vi "test_null_map.vi"() -> ()   [LabVIEW 2009]
doc: "Copyright (C) 2009, Stepan A. Baranov\nweb: http://www.OCTLab.org/\nemail: stepan@baranov.su"
uses:
  OCTLib.dll
panel:
  out "error out":errorcluster
  out "radius":i32
  out "width":i32
  out "height":i32
  in  "Small/Big":bool
  out "loop #":i32
  out "RSM_STAT time":u32
  out "LabView time":u32
  out "RSM_STAT Array":dbl[][](array[numeric])
  out "LabView Array":dbl[][](array[numeric])
  in  "stop":bool
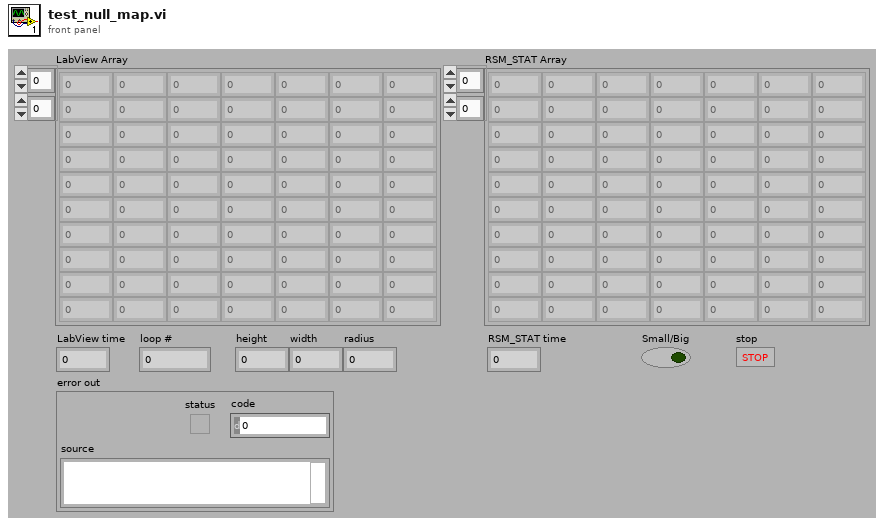
[diagram p1: front panel]
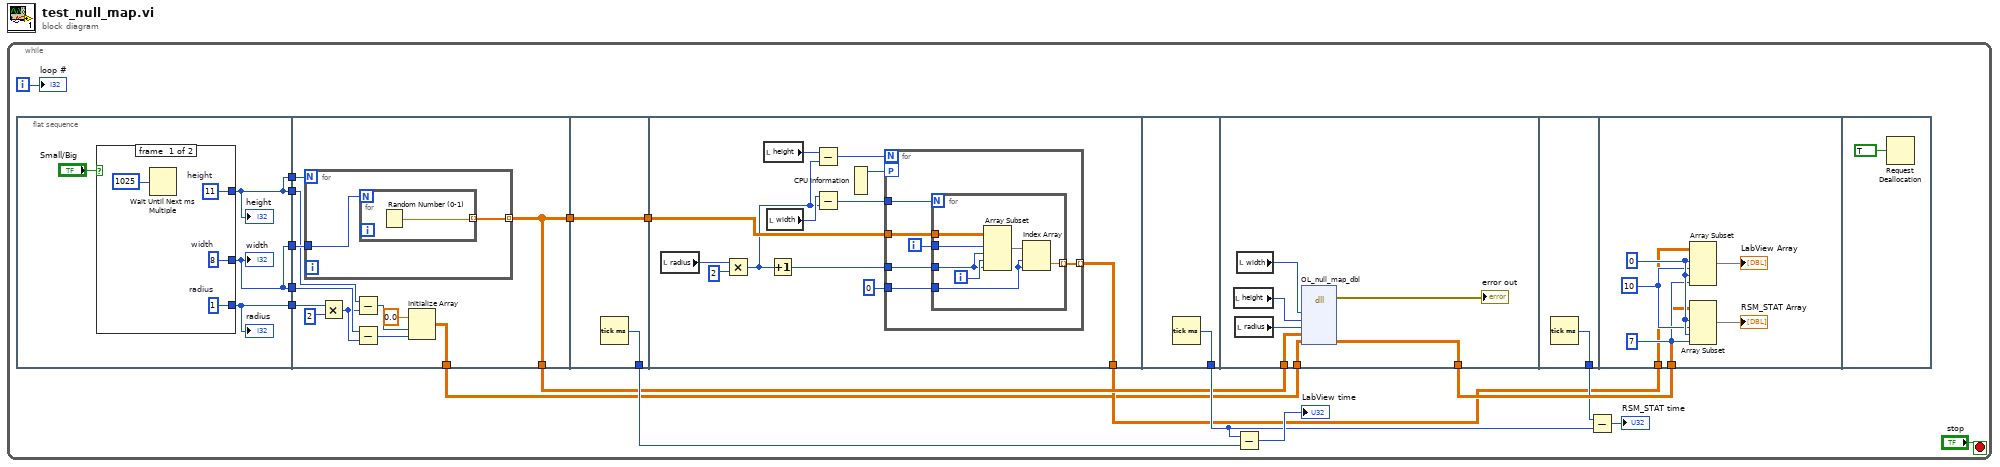
[diagram p0: block diagram]
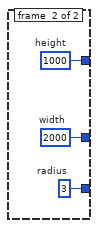
[diagram p2: hidden frame]
diagram:
  n1 = while {
    i -> [w11]
    stop <- "stop" stop-if-true
    n2 = flat-sequence {
      tunnel: [w19] -> w7
      tunnel: [w20] -> w6
      tunnel: [w21] -> w4
      tunnel: [w20] -> w3
      tunnel: [w19] -> w2
      tunnel: [w39] -> w10
      tunnel: [w39] -> w8
      tunnel: w7 -> [w41]
      tunnel: w6 -> [w40]
      tunnel: w4 -> [w37]
      tunnel: w3 -> [w35]
      tunnel: w2 -> [w33]
      tunnel: [w30] -> w1
      tunnel: [w46] -> w16
      tunnel: [w45] -> w9
      tunnel: w8 -> [w45]
      tunnel: w9 -> [w58]
      tunnel: [w47] -> w5
      tunnel: [w72] -> w13
      tunnel: w10 -> [w78]
      tunnel: [w77] -> w17
      tunnel: w1 -> [w79]
      tunnel: [w80] -> w14
      tunnel: w17 -> [w83]
      tunnel: w5 -> [w82]
      frame #0 {
        n3 = case shown="True" "Small/Big" {
          tunnel: [w24 w29] -> w20
          tunnel: [w25 w28] -> w19
          tunnel: [w26 w27] -> w21
          frame #0 {
            w26 = 1  # radius
            w25 = 8  # width
            w24 = 11  # height
            n4 = Wait Until Next ms Multiple(millisecond multiple=u32 1025) -> ()  [unwired: 1 out]
          }
          frame #1 {
            w27 = 3  # radius
            w28 = 2000  # width
            w29 = 1000  # height
          }
        }
        "height" <- w20
        "width" <- w19
        "radius" <- w21
      }
      frame #1 {
        n5 = for {
          N: w40 -> [_]
          tunnel: w41 -> [w43]
          tunnel: [w42] -> w39 mode=indexing
          n6 = for {
            N: w43 -> [_]
            tunnel: [w44] -> w42 mode=indexing
            n7 = Random Number (0-1)() -> (number: 0 to 1=w44:dbl)
          }
        }
        n8 = Multiply(x=w37, y=2) -> (x*y=w32:i32)
        n9 = Subtract(x=w35, y=w32) -> (x-y=w34:i32)
        n10 = Subtract(x=w33, y=w32) -> (x-y=w31:i32)
        n11 = Initialize Array(0.0 ("element"), w34, w31) -> (w30:dbl[][])
      }
      frame #2 {
        n12 = Tick Count (ms)() -> (millisecond timer value=w46:u32)
      }
      frame #3 {
        n13 = local read "radius"() -> (w57:i32)
        n14 = Multiply(x=w57, y=2) -> (x*y=w51:i32)
        n15 = local read "height"() -> (w54:i32)
        n16 = local read "width"() -> (w52:i32)
        n17 = Increment(x=w51) -> (x+1=w55:i32)
        n18 = Subtract(x=w54, y=w51) -> (x-y=w53:i32)
        n19 = Subtract(x=w52, y=w51) -> (x-y=w50:i32)
        n20 = CPU Information() -> (4:w49:i32)  [unwired: 3 out]
        n21 = for {
          N: w53 -> [_]
          tunnel: w58 -> [w63]
          tunnel: w55 -> [w62]
          tunnel: w50 -> [w61]
          workers-P: w49 -> [_]
          tunnel: 0 ("index") -> [w60]
          tunnel: [w59] -> w47 mode=indexing
          i -> [w64]
          n22 = for {
            N: w61 -> [_]
            tunnel: w64 -> [w71]
            tunnel: w63 -> [w69]
            tunnel: w62 -> [w68]
            tunnel: w60 -> [w66]
            tunnel: [w65] -> w59 mode=indexing
            i -> [w70]
            n23 = Array Subset(array=w69, index (row)=w71, length (row)=w68, index (col)=w70, length (col)=w68) -> (w67:dbl[][])
            n24 = Index Array(array=w67, index (row)=w66, index (col)=w66) -> (element=w65:dbl)
          }
        }
      }
      frame #4 {
        n25 = Tick Count (ms)() -> (millisecond timer value=w72:u32)
      }
      frame #5 {
        n26 = local read "height"() -> (w75:i32)
        n27 = local read "radius"() -> (w74:i32)
        n28 = local read "width"() -> (w76:i32)
        n29 = dll-call lib="OCTLib.dll" fn="OL_null_map_dbl"("width"=w76, "height"=w75, "radius"=w74, "input"=w78, "output"=w79) -> (error out=→"error out":errorcluster, "output"=w77:dbl[][])  [unwired: 8 in, 1 out]
      }
      frame #6 {
        n30 = Tick Count (ms)() -> (millisecond timer value=w80:u32)
      }
      frame #7 {
        w86 = 10 ("length")
        w85 = 7 ("length")
        w87 = 0 ("index")
        n31 = Array Subset(array=w82, index (row)=w87, length (row)=w86, index (col)=w87, length (col)=w85) -> (→"LabView Array":dbl[][])
        n32 = Array Subset(array=w83, index (row)=w87, length (row)=w86, index (col)=w87, length (col)=w85) -> (→"RSM_STAT Array":dbl[][])
      }
      frame #8 {
        n33 = Request Deallocation(TRUE ("flag")) -> ()
      }
    }
    n34 = Subtract(x=w13, y=w16) -> (x-y=→"LabView time":u32)
    n35 = Subtract(x=w14, y=w13) -> (x-y=→"RSM_STAT time":u32)
    "loop #" <- w11
  }
